vi "getStatus.vi"(8 "error in (no error)":errorcluster, 11 "Monochromator in":refnum<class "Monochromator.lvclass">) -> (0 "error out":errorcluster, 3 "Monochromator out":refnum<class "Monochromator.lvclass">)   [LabVIEW 2016, in "Monochromator.lvclass"]
uses:
  Monochromator.lvclass
  Monochromator.lvclass/Monochromator.ctl
  MonoStates/MonoState/MonoState.lvclass
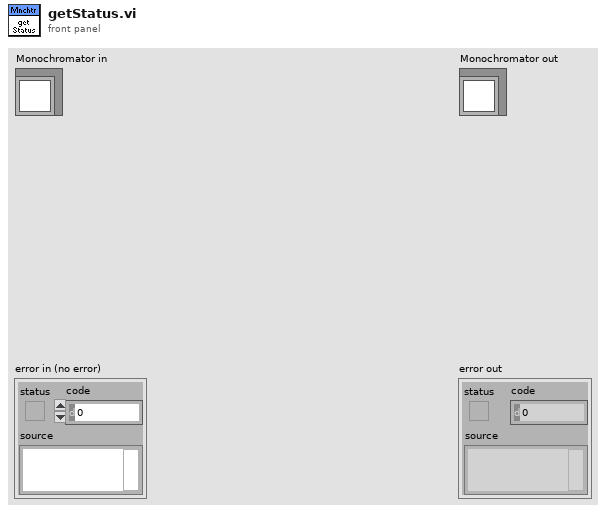
[diagram p1: front panel]
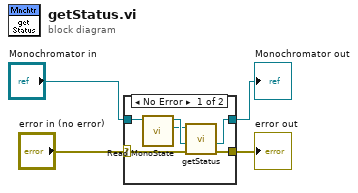
[diagram p0: block diagram]
diagram:
  n1 = case shown="No Error" "error in (no error)" {
    selector: "error in (no error)" -> [w9 w12]
    tunnel: [w8 w12] -> w1
    tunnel: [w7 w11] -> w3
    tunnel: "Monochromator in" -> [w10 w11]
    frame No Error {
      n2 = call "Read MonoState.vi"("Monochromator in"=w10) -> ("MonoState.lvclass"=w5:refnum<class "MonoState.lvclass">, "Monochromator out"=w6:refnum<class "Monochromator.lvclass">)  [unwired: 8 in, 1 out]
      n3 = call-dynamic "getStatus.vi"("error in (no error)"=w9, "Monochromator in"=w6, "MonoState in"=w5) -> ("error out"=w8:errorcluster, "Monochromator out"=w7:refnum<class "Monochromator.lvclass">)  [unwired: 6 in, 1 out]
    }
    frame Error {
    }
  }
  "error out" <- w1
  "Monochromator out" <- w3
